vi "Scintillator IDs.vi"() -> ()   [LabVIEW 2016]
panel:
  in  "Top layer IDs":i8[](array[numeric])=[8, 9, 10, 11, 12, 13, 14, 15]
  in  "Bottom layer IDs":i8[](array[numeric])=[0, 1, 2, 3, 4, 5, 6, 7]
  in  "Bottom layer Secondary IDs":i8[](array[numeric])=[4, 5, 6, 7]
  in  "Bottom layer Primary IDs":i8[](array[numeric])=[0, 1, 2, 3]
  in  "Top layer Secondary IDs":i8[](array[numeric])=[12, 13, 14, 15]
  in  "Top layer Primary IDs":i8[](array[numeric])=[8, 9, 10, 11]
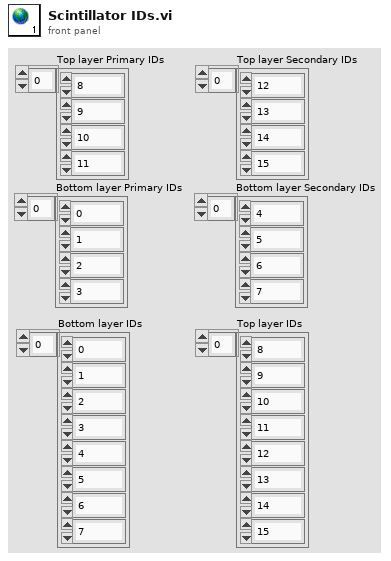
[diagram p1: front panel]
diagram:
